vi "Adapt to inputs.vi"(3 "Term Types":T1[](array[typedef]), 4 "XRef":refnum<vi>, 5 "State In":T4) -> (0 "Reply":string[](array[string]), 2 "State Out":T4)   [LabVIEW 2018, in "FilterArray.xnode"]
uses:
  FilterArray.xnode
  State.ctl
  <vilib>/XNodeSupport/XNodeTermTypeIDPair.ctl
  <vilib>/XNodeSupport/XNodeType.ctl
  <vilib>/XNodeSupport/XNodeString.ctl
  <userlib>/_LAVAcr/Scripting Tools/XNode Support/TypeDefs/Array element Tests.ctl
  <userlib>/_LAVAcr/Scripting Tools/XNode Support/XNode Support.lvlib
  <vilib>/XNodeSupport/NI_XNodeSupport.lvlib
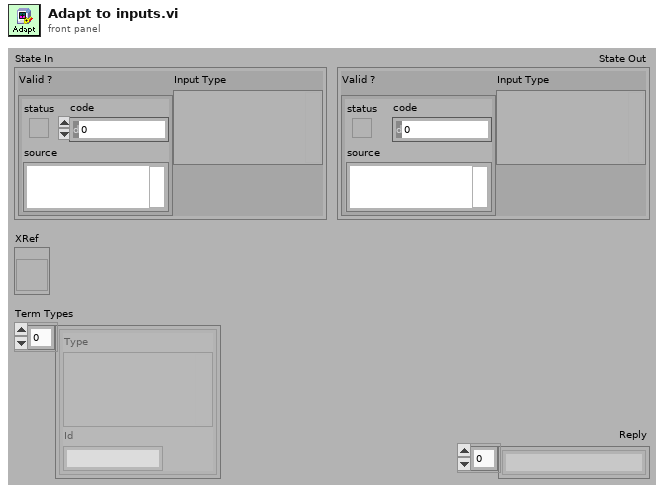
[diagram p1: front panel]
types:
  T1 = typedef "NI_XNodeSupport.lvlib/XNodeTermTypeIDPair.ctl" = cluster{"Type":T2, "Id":T3}
  T2 = typedef "NI_XNodeSupport.lvlib/XNodeType.ctl" = variant
  T3 = typedef "NI_XNodeSupport.lvlib/XNodeString.ctl" = string
  T4 = typedef "FilterArray.xnode/State.ctl" = cluster{"Valid ?":errorcluster, "Input Type":variant}
  T5 = typedef "Scripting Tools.lvlib/XNode Support.lvlib/Array element Tests.ctl" = enum16{"Any Element", "Numeric", "Integer", "Float", "Complex", "Boolean", "String", "Sortable"}
  T6 = enum16{"No Check", "At Least n dimensions", "Exactly N Dimensions"}
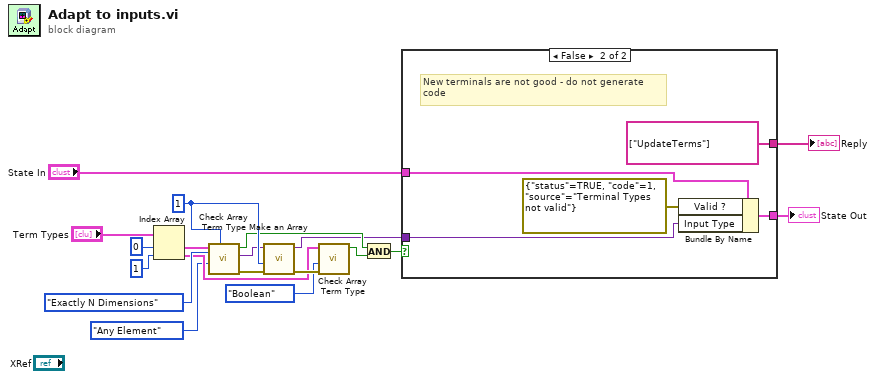
[diagram p0: block diagram]
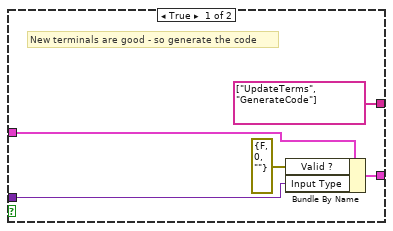
[diagram p2: hidden frame]
diagram:
  w12 = 1 ("Dimensions Required")
  n1 = Index Array(array="Term Types", index #1=0 ("Dimension"), index #2=1 ("index")) -> (element #1=w14:T1, element #2=w10:T1)
  n2 = call <userlib>:"Check Array Term Type.vi"("Dimensions Required"=w12, "Element Check"=Array_element_Tests."Any Element", "Dimension Check"=T6."Exactly N Dimensions", "Term Type"=w14) -> ("error out"=w4:errorcluster, "Element Type"=w5:variant, "Is Good ?"=w3:bool)  [unwired: 1 in, 4 out]
  n3 = call <userlib>:"Make an Array.vi"("error in (no error)"=w4, "Number of Dimensions"=w12, "Element Type"=w5) -> ("error out"=w11:errorcluster, "Array Type"=w1:variant)  [unwired: 7 out]
  n4 = call <userlib>:"Check Array Term Type.vi"("error in (no error)"=w11, "Element Check"=Array_element_Tests."Boolean", "Term Type"=w10) -> ("Is Good ?"=w2:bool)  [unwired: 2 in, 6 out]
  n5 = And(x=w3, y=w2) -> (x .and. y?=w7:bool)
  n6 = case shown="False" w7 {
    tunnel: "State In" -> [w24 w29]
    tunnel: [w22 w27] -> w18
    tunnel: [string[] ["UpdateTerms", "GenerateCode"] ("Reply") string[] ["UpdateTerms"] ("Reply")] -> w17
    tunnel: w1 -> [w20 w25]
    frame True {
      # "New terminals are good - so generate the code"
      n7 = Bundle By Name(cluster=w24, "Valid ?"=errorcluster {"status"=FALSE, "code"=0, "source"=""}, "Input Type"=w20) -> (w22:T4)
    }
    frame False {
      # "New terminals are not good - do not generate\ncode"
      n8 = Bundle By Name(cluster=w29, "Valid ?"=errorcluster {"status"=TRUE, "code"=1, "source"="Terminal Types not valid"}, "Input Type"=w25) -> (w27:T4)
    }
  }
  "Reply" <- w17
  "State Out" <- w18
